vi "例4-36.vi"() -> ()   [LabVIEW 2019]
uses:
  <vilib>/Native 3D Graph/xcontrol/3DPC_SurfacePlot.xctl
panel:
  out "3D Graph":refnum<class "Base Datatype.lvclass">[](xcontrol) caption="三维图形"
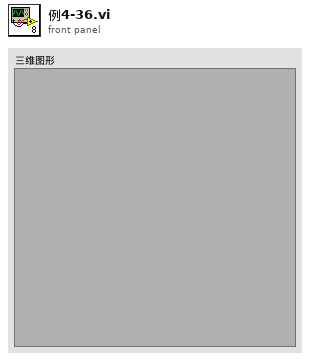
[diagram p1: front panel]
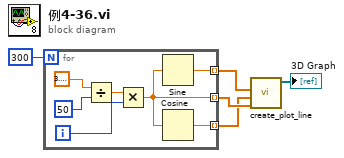
[diagram p0: block diagram]
diagram:
  n1 = for {
    N: 300 -> [_]
    tunnel: [w8] -> w3 mode=indexing
    tunnel: [w7] -> w2 mode=indexing
    tunnel: [w6] -> w1 mode=indexing
    i -> [w9]
    n2 = Divide(x=3.141592653589793, y=50) -> (x/y=w10:dbl)
    n3 = Multiply(x=w10, y=w9) -> (x*y=w8:dbl)
    n4 = Sine(x=w8) -> (sin(x)=w6:dbl)
    n5 = Cosine(x=w8) -> (cos(x)=w7:dbl)
  }
  n6 = call <vilib>:"create_plot_line.vi"("z vector"=w3, "y vector"=w2, "x vector"=w1) -> ("plots out"=→"3D Graph":refnum<class "Base Datatype.lvclass">[])  [unwired: 2 in, 6 out]
